vi "HEWH Extract At Index.vi"(8 "Error In":errorcluster, 10 "Test Start Index in":i32, 11 "all rows in":string[][](array[string])) -> (0 "Error Out":errorcluster, 2 "Test Start Index out":i32, 3 "Array":string[][](array[string]))   [LabVIEW 2016]
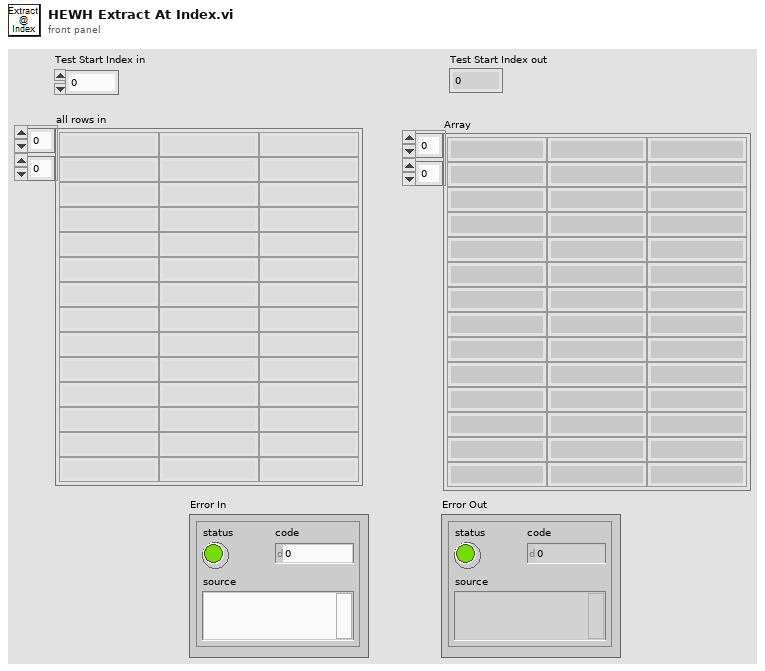
[diagram p1: front panel]
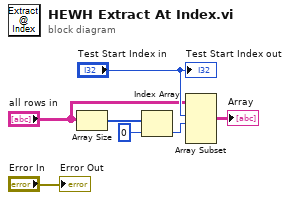
[diagram p0: block diagram]
diagram:
  n1 = Array Size(array="all rows in") -> (size(s)=w2:i32[])
  n2 = Index Array(array=w2, index=0) -> (element=w5:i32)
  n3 = Array Subset(array="all rows in", index (row)="Test Start Index in", length (row)=w5) -> (→"Array":string[][])  [unwired: 2 in]
  "Test Start Index out" <- "Test Start Index in"
  "Error Out" <- "Error In"
